vi "Create.vi"(8 "error in (no error)":errorcluster, 11 "Super Resolution Model Directory (Default: Not A Path)":path=path "") -> (0 "error out":errorcluster, 3 "New Barcode Detector":refnum<class "Barcode Detector.lvclass">)   [LabVIEW 2020, in "g_ar_toolkit.feature_detection.lvlib" / "Barcode Detector.lvclass"]
uses:
  Barcode Detector.lvclass
  Barcode Detector.lvclass/Barcode Detector.ctl
  g_ar_toolkit.common/g_ar_toolkit.common.lvlib
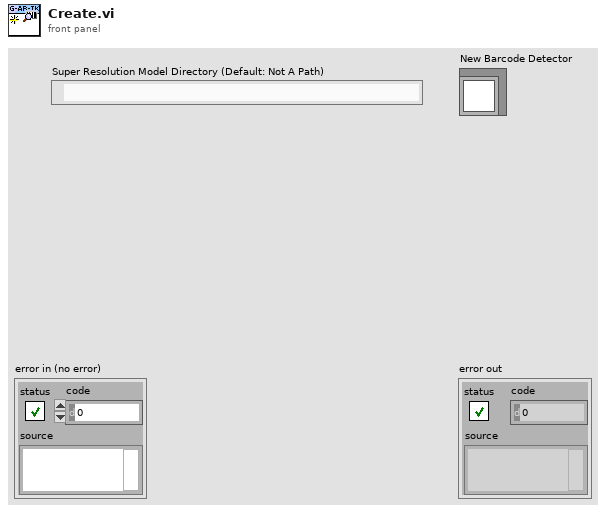
[diagram p1: front panel]
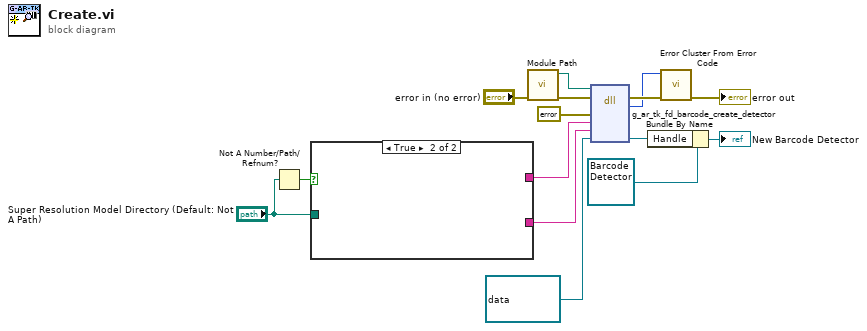
[diagram p0: block diagram]
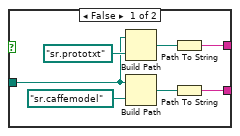
[diagram p2: hidden frame]
diagram:
  n1 = Not A Number/Path/Refnum?(number/path/refnum="Super Resolution Model Directory (Default: Not A Path)") -> (NaN/Path/Refnum?=w3:bool)
  n2 = case shown="True" w3 {
    tunnel: [w22 _] -> w12
    tunnel: [w21 _] -> w11
    tunnel: "Super Resolution Model Directory (Default: Not A Path)" -> [w16 _]
    frame False {
      n3 = Build Path(base path=w16, name or relative path=path "sr.prototxt" ("Filepath")) -> (appended path=w19:path)
      n4 = Build Path(base path=w16, name or relative path=path "sr.caffemodel" ("Filepath")) -> (appended path=w17:path)
      n5 = Path To String(path=w19) -> (string=w22:string)
      n6 = Path To String(path=w17) -> (string=w21:string)
    }
    frame True {
    }
  }
  n7 = call "Module Path.vi"("error in (no error)"="error in (no error)") -> ("error out"=w2:errorcluster, "Path"=w1:path)  [unwired: 9 in]
  n8 = dll-call lib="?" fn="g_ar_tk_fd_barcode_create_detector" ("g_ar_toolkit.*.*:g_ar_tk_capture_context_create")(path in=w1, error in=w2, "error_cluster"=errorcluster {"status"=FALSE, "code"=0, "source"=""} ("error constant"), "proto_path"=w12, "model_path"=w11, "EDVR"=refnum<data-value> refnum) -> (error out=w10:errorcluster, "MgErr"=w6:i32, "EDVR"=w8:refnum<data-value>)  [unwired: 4 in, 1 out]
  n9 = Bundle By Name(cluster=refnum<class "Barcode Detector.lvclass"> refnum ("Barcode Detector in"), "Handle"=w8) -> (→"New Barcode Detector":refnum<class "Barcode Detector.lvclass">)
  n10 = call <vilib>:"Error Cluster From Error Code.vi"("error in (no error)"=w10, "error code (0)"=w6) -> ("error out"=→"error out":errorcluster)  [unwired: 7 in]
